vi "SM_S700_Serial_String_#MS.vi"(8 "error in (no error)":errorcluster, 11 "read buffer":string) -> (0 "error out":errorcluster, 1 "ch4":dbl, 2 "co2":dbl, 3 "timestamp":timestamp, 5 "h2":dbl)   [LabVIEW 2011]
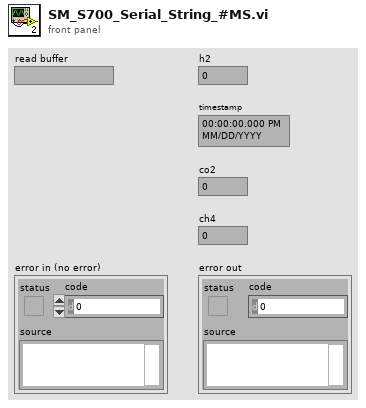
[diagram p1: front panel]
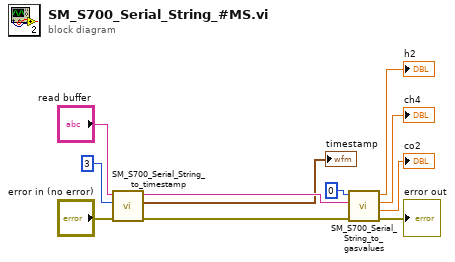
[diagram p0: block diagram]
diagram:
  n1 = call "SM_S700_Serial_String_to_timestamp.vi"("error in (no error)"="error in (no error)", "initial scan location"=u32 3, "read buffer"="read buffer") -> ("error out"=w5:errorcluster, "Time Stamp"=→"timestamp":timestamp, "String"=w4:string)  [unwired: 6 in]
  n2 = call "SM_S700_Serial_String_to_gasvalues.vi"("error in (no error)"=w5, "String"=w4, "initial scan location in"=u32 0 ("initial scan location 2")) -> ("error out"=→"error out":errorcluster, "co2"=→"co2":dbl, "ch4"=→"ch4":dbl, "h2"=→"h2":dbl)  [unwired: 5 in]
